vi "Match Meta.vi"(8 "error in (no error)":errorcluster, 9 "Meta":T1[](array[typedef]), 10 "Element":refnum<class "Config Element.lvclass">) -> (0 "error out":errorcluster, 2 "Match":bool)   [LabVIEW 2020, in "CDM-Config.lvlib" / "Config Manager.lvclass"]
uses:
  Config Manager.lvclass
  Config Element/Config Element.lvclass
  Meta Data.ctl
  b47f34b2-d53d-48ea-85ed-16fae7f57de2.vi
  <vilib>/Comparison/Equal/Equal Functor/Equal Functor.lvclass
  CDM-Config.lvlib
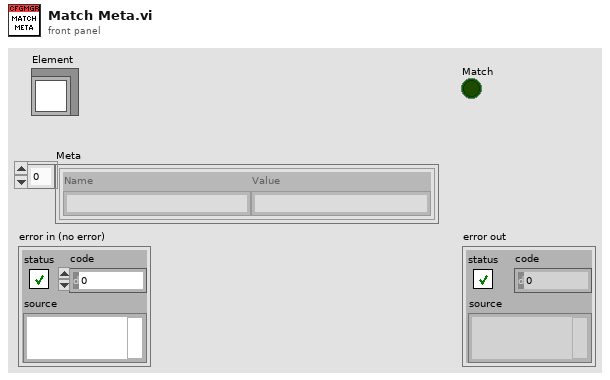
[diagram p1: front panel]
types:
  T1 = typedef "CDM-Config.lvlib/Meta Data.ctl" = cluster{"Name":string, "Value":string}
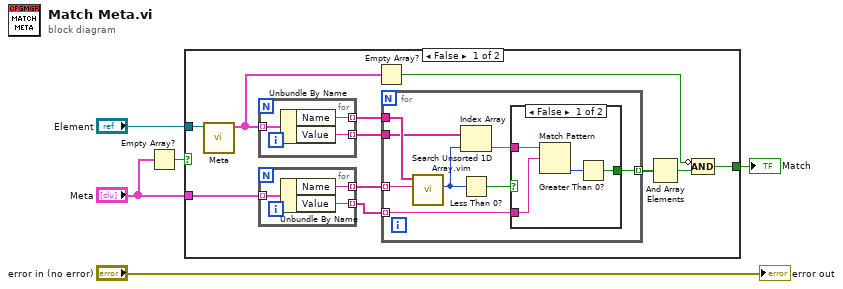
[diagram p0: block diagram]
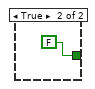
[diagram p2: hidden frame]
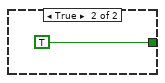
[diagram p3: hidden frame]
diagram:
  n1 = Empty Array?(array="Meta") -> (empty?=w2:bool)
  n2 = case shown="False" w2 {
    tunnel: "Element" -> [w16 _]
    tunnel: "Meta" -> [w13 _]
    tunnel: [w7 TRUE] -> w1
    frame False {
      n3 = call "Meta.vi"("Config Element in"=w16) -> ("Meta Data"=w8:T1[])  [unwired: 9 in, 1 out]
      n4 = for {
        tunnel: w8 -> [w22] mode=indexing
        tunnel: [w21] -> w9 mode=indexing
        tunnel: [w20] -> w12 mode=indexing
        n5 = Unbundle By Name(w22) -> ("Name"=w21:string, "Value"=w20:string)
      }
      n6 = for {
        tunnel: w13 -> [w19] mode=indexing
        tunnel: [w18] -> w15 mode=indexing
        tunnel: [w17] -> w14 mode=indexing
        n7 = Unbundle By Name(w19) -> ("Name"=w18:string, "Value"=w17:string)
      }
      n8 = Empty Array?(array=w8) -> (empty?=w6:bool)
      n9 = for {
        tunnel: w15 -> [w29] mode=indexing
        tunnel: w9 -> [w28]
        tunnel: w12 -> [w25]
        tunnel: w14 -> [w23] mode=indexing
        tunnel: [w26] -> w11 mode=indexing
        n10 = call "Search Unsorted 1D Array.vim"("element"=w29, "unsorted 1D array"=w28) -> ("index of element"=w30:i32)  [unwired: 9 in]
        n11 = Index Array(array=w25, index=w30) -> (element=w24:string)
        n12 = Less Than 0?(x=w30) -> (x < 0?=w27:bool)
        n13 = case shown="False" w27 {
          tunnel: w23 -> [w33 _]
          tunnel: w24 -> [w34 _]
          tunnel: [w31 FALSE] -> w26
          frame False {
            n14 = Match Pattern(string=w34, regular expression=w33) -> (offset past match=w32:i32)  [unwired: 1 in, 3 out]
            n15 = Greater Than 0?(x=w32) -> (x > 0?=w31:bool)
          }
          frame True {
          }
        }
      }
      n16 = And Array Elements(Boolean array=w11) -> (logical AND=w10:bool)
      n17 = Compound Arithmetic op=AND(invert w6, w10) -> (w7:bool)
    }
    frame True {
    }
  }
  "Match" <- w1
  "error out" <- "error in (no error)"
